vi "datatojson.vi"(8 "error in (no error)":errorcluster caption="错误输入（无错误）", 11 "HTTP发送 输入":refnum<class "HTTP发送.lvclass">) -> (0 "error out":errorcluster caption="错误输出", 3 "HTTP发送 输出":refnum<class "HTTP发送.lvclass">)   [LabVIEW 2022 SP3, in "工况数据上传.lvlib" / "HTTP发送.lvclass"]
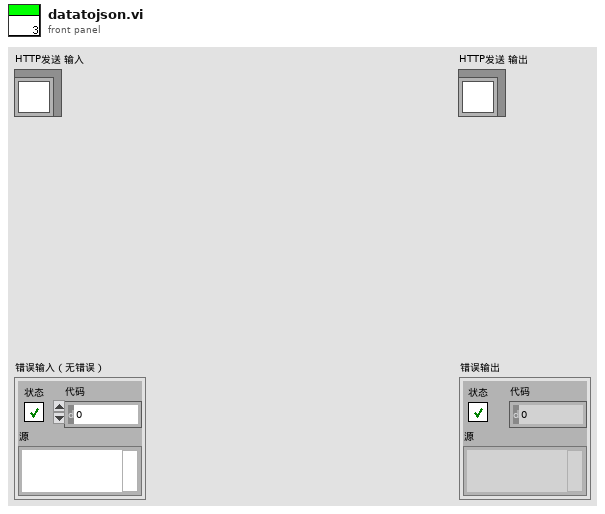
[diagram p1: front panel]
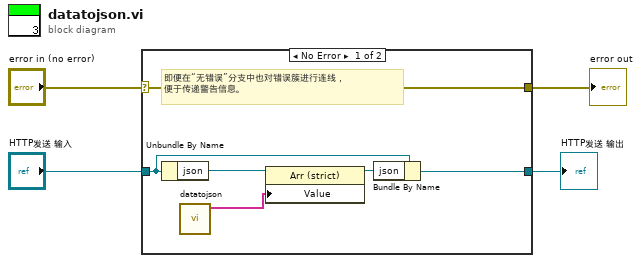
[diagram p0: block diagram]
diagram:
  n1 = case shown="No Error" "error in (no error)" {
    selector: "error in (no error)" -> [w10 w12]
    tunnel: [w10 w12] -> w3
    tunnel: [w5 w11] -> w1
    tunnel: "HTTP发送 输入" -> [w7 w11]
    frame No Error {
      # "即便在“无错误”分支中也对错误簇进行连线，\n便于传递警告信息。"
      n2 = Unbundle By Name(w7) -> ("json"=w9:refnum<vi>)
      n3 = call "datatojson.vi"() -> ("json"=w8:string[])  [unwired: 11 in]
      n4 = property class="Arr (strict)"(reference=w9, "Value"=w8) -> (reference out=w6:refnum<vi>)  [unwired: 1 in, 1 out]
      n5 = Bundle By Name(cluster=w7, "json"=w6) -> (w5:refnum<class "HTTP发送.lvclass">)
    }
    frame Error {
    }
  }
  "error out" <- w3
  "HTTP发送 输出" <- w1
